vi "HMI GV.vi"() -> ()   [LabVIEW 2021]
panel:
  in  "Connected?":bool
  out "writer endpoint":refnum<k21>
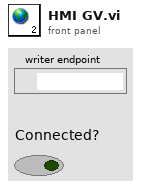
[diagram p1: front panel]
diagram:
